vi "Entry.vi"(8 "error in (no error)":errorcluster, 11 "New State":refnum<class "Connected.lvclass">) -> (0 "error out":errorcluster, 3 "State out":refnum<class "Connected.lvclass">)   [LabVIEW 2013, in "Receiver.lvlib" / "Receive Commands Using State Actors.lvlib" / "Connect Command.lvlib" / "Executing States.lvlib" / "Connected.lvclass"]
doc: "This is an abstract method. Override this method to define the behavior when you enter the state."
uses:
  Connected.lvclass
  Executing State.lvclass
  <vilib>/ActorFramework/Actor/Actor.lvclass/Actor.ctl
  <vilib>/ActorFramework/Message Enqueuer/Message Enqueuer.lvclass/Message Enqueuer.ctl
  <vilib>/ActorFramework/Message Enqueuer/Init from Existing Queue.vi
  <vilib>/ActorFramework/Message Enqueuer/Enqueue.vi
  <vilib>/ActorFramework/Message Priority Queue/Priority Enqueue.vi
  <vilib>/ActorFramework/Message Enqueuer/Message Enqueuer.lvclass
  Command Messages/Complete Command Msg/Complete Command Msg.lvclass
  <vilib>/ActorFramework/Actor/Actor.lvclass
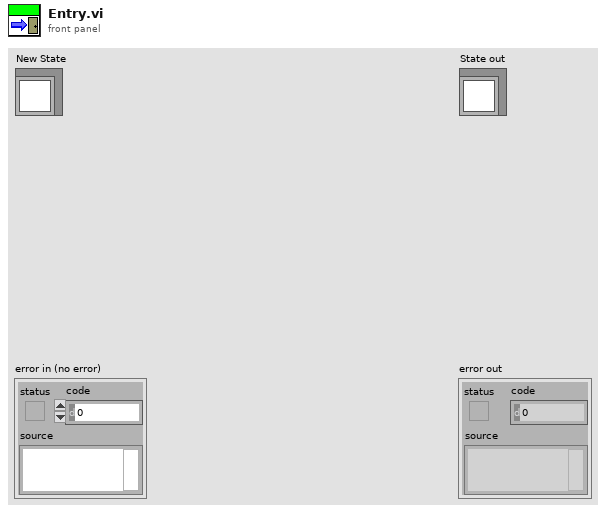
[diagram p1: front panel]
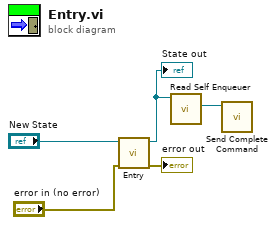
[diagram p0: block diagram]
diagram:
  n1 = call-parent "Entry.vi"("error in (no error)"="error in (no error)", "New State"="New State") -> ("error out"=→"error out":errorcluster, "State out"=w2:refnum<class "Connected.lvclass">)  [unwired: 8 in]
  "State out" <- w2
  n2 = call <vilib>:"Read Self Enqueuer.vi"("Actor"=w2) -> ("Self Enqueuer"=w3:refnum<class "Message Enqueuer.lvclass">)  [unwired: 10 in]
  n3 = call "Send Complete Command.vi"("Message Enqueuer"=w3) -> ()  [unwired: 9 in, 2 out]
